vi "数据处理3.vi"(6 "原始数据文件名":string, 7 "去噪信号保存的文件名":string, 9 "数组中的数据（输入）":dbl[](array[numeric])) -> (1 "字符串（输出）":string, 2 "特征值（输出）":dbl[][](array[numeric]), 3 "去噪后波形图":dbl[][](graph))   [LabVIEW 2018]
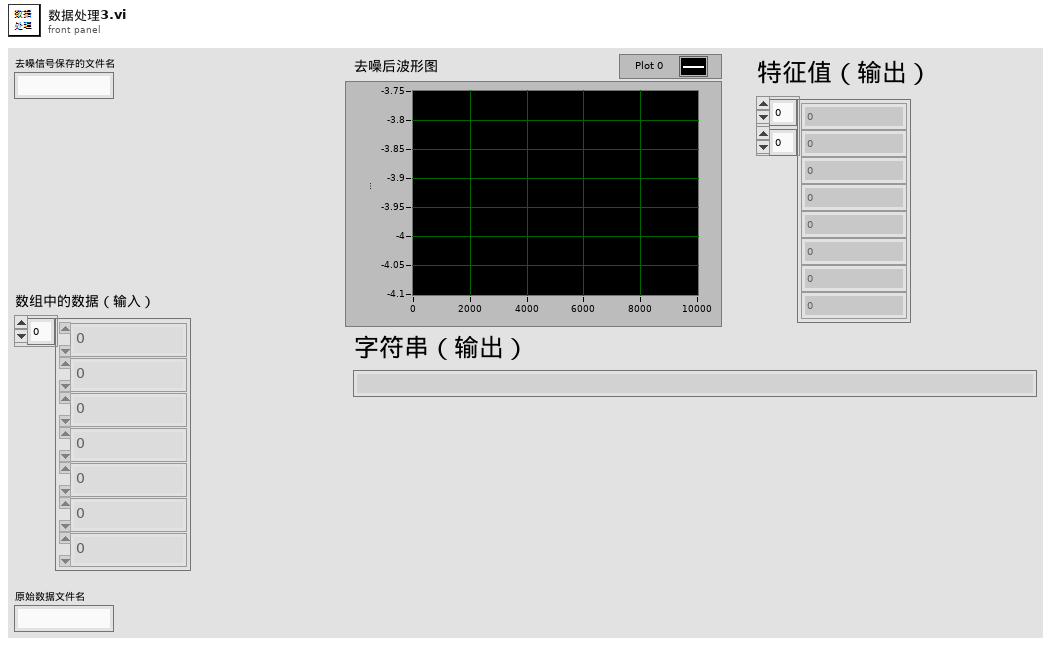
[diagram p1: front panel]
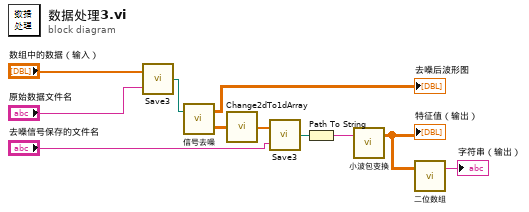
[diagram p0: block diagram]
diagram:
  n1 = call "Save3.vi"("要保存的文件名（输入）"="原始数据文件名", "数组中的数据（输入）"="数组中的数据（输入）") -> ("文件保存路径（输出）"=w10:path)
  n2 = call "信号去噪.vi"("文件路径（输入）"=w10) -> ("去噪后数据输出"=w6:dbl[][], "去噪后波形图（输出）"=→"去噪后波形图":dbl[][])  [unwired: 1 in]
  n3 = call "Change2dTo1dArray.vi"("AI2去噪后数据"=w6) -> ("AI2一维数组"=w5:dbl[])
  n4 = call "Save3.vi"("要保存的文件名（输入）"="去噪信号保存的文件名", "数组中的数据（输入）"=w5) -> ("文件保存路径（输出）"=w8:path)
  n5 = Path To String(path=w8) -> (string=w7:string)
  n6 = call "小波包变换.vi"("数据文件路径（输入）"=w7) -> ("特征值（输出）"=w3:dbl[][])  [unwired: 2 in]
  "特征值（输出）" <- w3
  n7 = call "二位数组.vi"("二位数组（输入）"=w3) -> ("字符串（输出）"=→"字符串（输出）":string)  [unwired: 1 in, 1 out]
